vi "RS32.vi"(2 "R":u32 format="%x", 3 "S":u32 format="%x") -> (0 "~Q":u32=4294967295 format="%x", 1 "Q":u32 format="%x")   [LabVIEW 2019, in "Triggers.lvlib"]
uses:
  Triggers.lvlib
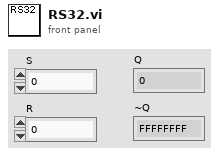
[diagram p1: front panel]
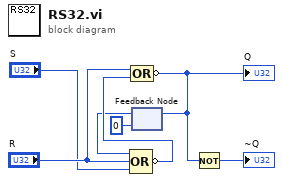
[diagram p0: block diagram]
diagram:
  n1 = feedback #1(u32 0) -> (w4:u32)
  n2 = Compound Arithmetic op=OR(w4, "R", "S") -> (invert w6:u32)
  n3 = Compound Arithmetic op=OR("R", w6) -> (invert w3:u32)
  "Q" <- w3
  n4 = feedback-in #1(w3) -> ()
  n5 = Not(x=w3) -> (.not. x?=→"~Q":u32)
